vi "web_test.vi"() -> ()   [LabVIEW 2009]
panel:
  in  "stop":bool
  out "Numeric":dbl=6.2863058325034915
  in  "Delay (ms)":dbl(slide)=682.8571428571429 min=0.0 max=2000.0 step=100.0 scale=100.0..1000.0
  out "Meter":dbl(knob)=6.2863058325034915 scale=0.0..100.0
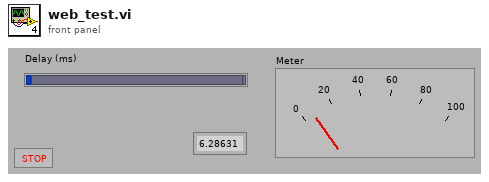
[diagram p1: front panel]
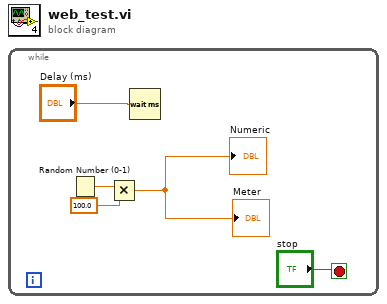
[diagram p0: block diagram]
diagram:
  n1 = while {
    stop <- "stop" stop-if-true
    n2 = Random Number (0-1)() -> (number: 0 to 1=w4:dbl)
    n3 = Multiply(x=w4, y=100.0) -> (x*y=→"Meter" →"Numeric":dbl)
    n4 = Wait (ms)(milliseconds to wait="Delay (ms)") -> ()  [unwired: 1 out]
  }
